vi "Enum to Expected Boolean Array.vi"(0 "reference":refnum<vi>, 7 "index":i32, 11 "error in (no error)":errorcluster) -> (4 "Enum Names":string[](array[string]), 8 "Expected Bool Array":bool[](array[boolean]), 15 "error out":errorcluster)   [LabVIEW 2016, in "Centauro.lvlib"]
uses:
  Projects/Centauro.lvlib
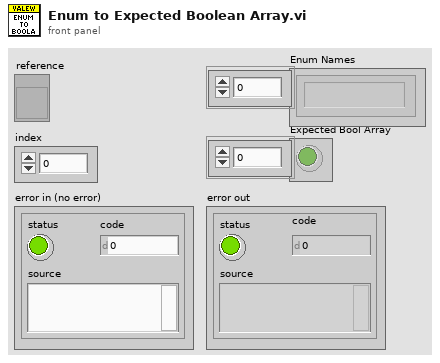
[diagram p1: front panel]
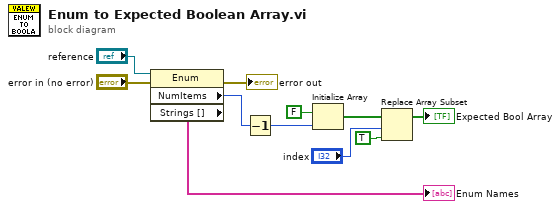
[diagram p0: block diagram]
diagram:
  n1 = property class="Enum"(reference="reference", error in="error in (no error)") -> (error out=→"error out":errorcluster, "NumItems"=w10:u32, "Strings []"=→"Enum Names":string[])  [unwired: 1 out]
  n2 = Decrement(x=w10) -> (x-1=w9:u32)
  n3 = Initialize Array(FALSE, w9) -> (w8:bool[])
  n4 = Replace Array Subset(array=w8, new element=TRUE ("new element/subarray"), index="index") -> (→"Expected Bool Array":bool[])
